vi "Enumerate Plugins.vi"(8 "error in (no error)":errorcluster, 11 "Plugin in":refnum<class "Plugin.lvclass">) -> (0 "error out":errorcluster, 2 "Available Plugins":string[](array[string]), 3 "Plugin out":refnum<class "Plugin.lvclass">)   [LabVIEW 2020, in "neg-pkg.lvlib" / "Plugin.lvclass"]
uses:
  Plugin.lvclass
  <vilib>/regexp/Match Regular Expression.xnode
  neg-pkg.lvlib
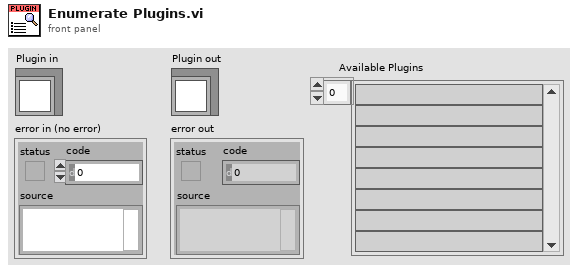
[diagram p1: front panel]
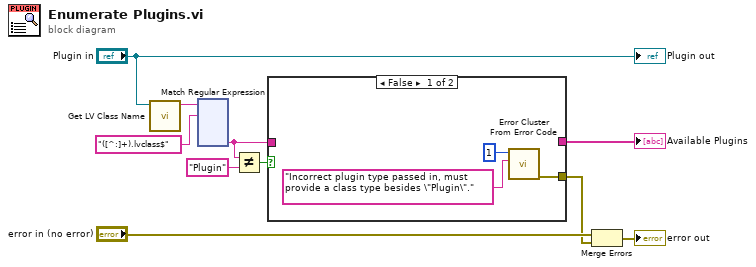
[diagram p0: block diagram]
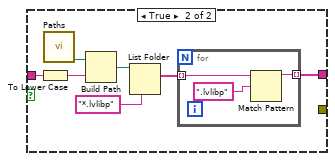
[diagram p2: hidden frame]
diagram:
  n1 = call <vilib>:"Get LV Class Name.vi"("object"="Plugin in") -> ("class name"=w9:string)  [unwired: 9 in, 1 out]
  n2 = xnode "Match Regular Expression"("input string"=w9, "regular expression"="([^:]+).lvclass$") -> ("submatch 1"=w5:string)  [unwired: 4 in, 5 out]
  n3 = Not Equal?(x=w5, y="Plugin") -> (x != y?=w3:bool)
  n4 = case shown="False" w3 {
    tunnel: w5 -> [_ w20]
    tunnel: [_ w14] -> w4
    tunnel: [w11 _] -> w1
    frame False {
      n5 = call <vilib>:"Error Cluster From Error Code.vi"("error message (\"\")"="Incorrect plugin type passed in, must provide a class type besides \"Plugin\".", "error code (0)"=1) -> ("error out"=w11:errorcluster)  [unwired: 7 in]
    }
    frame True {
      n6 = To Lower Case(string=w20) -> (all lower case string=w18:string)
      n7 = call "Paths.vi"() -> ("ppl Path"=w19:path)  [unwired: 8 in, 3 out]
      n8 = Build Path(base path=w19, name or relative path=w18) -> (appended path=w17:path)
      n9 = List Folder(path=w17, pattern="*.lvlibp") -> (filenames=w15:string[])  [unwired: 2 in, 3 out]
      n10 = for {
        tunnel: w15 -> [w23] mode=indexing
        tunnel: [w21] -> w14 mode=indexing
        n11 = Match Pattern(string=w23, regular expression=".lvlibp" ("substring (\"\")")) -> (before substring=w21:string)  [unwired: 1 in, 3 out]
      }
    }
  }
  "Available Plugins" <- w4
  n12 = Merge Errors("error in (no error)", w1) -> (→"error out":errorcluster)
  "Plugin out" <- "Plugin in"
